vi "ALL1.vi"   [LabVIEW 2016, in "Test2.lvrbt"]
uses:
  Test2.lvrbt
  <vilib>/NXT/Hardware/Plugins/Tetrix DC Motor/TetrixDCMotorAddress.ctl
  <vilib>/NXT/Hardware/Plugins/Tetrix 180 deg Servo/Tetrix180ServoAddress.ctl
  <vilib>/NXT/Block Support/NXT_InputPort.ctl
  <vilib>/NXT/Subs/ColorSensorColors.ctl
  <vilib>/NXT/NXTIO Xnodes/NXTIONodeSubVIs/TETRIX IO Move Servos.vi
  <vilib>/NXT/Dual Mode Library/Waits/Wait_Num.vi
  <vilib>/NXT/NXTIO Xnodes/NXTIONodeSubVIs/TETRIX IO Move DC Motors.vi
  <vilib>/NXT/NXTIO Xnodes/NXTIONodeSubVIs/TETRIX IO Stop DC Motors.vi
  <vilib>/NXT/Dual Mode Library/Waits/Wait_EV3_Ultrasonic_Centimeter_Closer.vi
  <vilib>/NXT/Dual Mode Library/Waits/Wait_EV3_Ultrasonic_Centimeters_Further.vi
  <vilib>/NXT/Dual Mode Library/Waits/Wait_Touch.vi
  <vilib>/NXT/Dual Mode Library/Waits/Wait_EV3_Color_Color.vi
  <vilib>/NXT/NXTIO Xnodes/AddressXNode/NXTIOAddress.xnode
  <vilib>/NXT/Subs/LVHSConnector.ctl
  <vilib>/NXT/NXTIO Xnodes/NXTIOXNode/NXTIO.xnode
  <vilib>/NXT/LegoClasses/BrickReference/BrickReference.lvclass
types:
  T1 = typedef "Tetrix180ServoAddress.ctl" = i32
  T2 = cluster{"Tetrix180Servo":T1, "Tetrix180Servo 2":T1, "Tetrix180Servo 3":T1, "Tetrix180Servo 4":T1, "Tetrix180Servo 5":T1, "Tetrix180Servo 6":T1}
  T3 = typedef "TetrixDCMotorAddress.ctl" = i32
  T4 = cluster{"TetrixDCMotor":T3, "TetrixDCMotor 2":T3}
  T5 = cluster{"Tetrix180Servo":T1, "Tetrix180Servo":T1, "Tetrix180Servo":T1, "Tetrix180Servo":T1, "Tetrix180Servo":T1, "Tetrix180Servo":T1}
  T6 = typedef "LVHSConnector.ctl" = refnum<class "BrickReference.lvclass">
  T7 = typedef "NXT_InputPort.ctl" = u32
  T8 = typedef "ColorSensorColors.ctl" = enum16{"No Color", "Black", "Blue", "Green", "Yellow", "Red", "White", "Brown"}
diagram:
  # "FILE: BACK TOBASE2\n\nTHE ROBOT WILL GO TO BASE"
  # "FILE: SAVETOUCH \n\nTHE ROBOT WILL DETECT THE RACK \nAND STRAIGHT THE POSITION"
  # "FILE: SAVETOUCH \n\nTHE ROBOT WILL DETECT THE RACK \nAND STRAIGHT THE POSITION"
  # "FILE: DETECT REFERENCE LINE, AFTER AIMING\n\nTHE ROBOT WILL GET A NEW POSITION AFTER LAUNCH THE BALL"
  # "FILE: LAUNCHFIRSTBALL\n\nTHE SECOND BALL WILL BE  LAUNCH"
  # "FILE: TRAPBALL\n\nTHE ROBOT WILL MOVE FOWARD TO TRAP THE BALL"
  # "FILE: GETSEECONDBALL\n\nTHE ROBOT WILL START TO DETECT AND PICKUP THE SECOND BALL"
  # "FILE: DETECT REFERENCE LINE, AFTER AIMING\n\nTHE ROBOT WILL GET A NEW POSITION AFTER LAUNCH THE BALL"
  # "FILE: LAUNCHFIRSTBALL\n\nTHE FIRST BALL WILL BE  LAUNCH"
  # "FILE: SERVOSETTING\n\nTHE FIRST BALL WILL BE PICKUP"
  # "FILE: DETECTFIRSTBALL\n\nTHE ROBOT WILL MOVE INFRONT TO DETECT THE FIRST BALL"
  # "FILE: SAVETOUCH \n\nTHE ROBOT WILL DETECT THE RACK \nAND STRAIGHT THE POSITION"
  # "FILE:  motor setting\n\nTHE ROBOT WILL MOVE OUT FROM THE BASE."
  n1 = flat-sequence {
    tunnel: [w13] -> w12
    frame #0 {
      n2 = xnode "Motors"() -> ("Motor"=w22:T5)
      n3 = xnode "Move Servos"("Position 6"=u8 8, "Position 5"=u8 237, "Position 4"=u8 40, "Position 3"=u8 7, "Position 2"=u8 0, "Position 1"=u8 220, "Motors"=w22) -> ("NXT/EV3"=w15:T6)  [unwired: 1 in]
      n4 = xnode "Motors"() -> ("Motor"=w27:cluster{"TetrixDCMotor":T3, "TetrixDCMotor":T3})
      n5 = call-poly <vilib>:"PolyWait.vi"("Time (1 sec)"=sgl 1.0, "NXT/EV3"=w15) -> ("NXT/EV3"=w14:T6)  [unwired: 2 in]
      n6 = xnode "Move Motors"("Power/Speed 2"=i8 50, "Power/Speed 1"=i8 51, "Motors"=w27, "NXT/EV3"=w14) -> ("NXT/EV3"=w30:T6)
      n7 = call-poly <vilib>:"PolyWait.vi"("Time (1 sec)"=sgl 2.0, "NXT/EV3"=w30) -> ("NXT/EV3"=w28:T6)  [unwired: 2 in]
      n8 = xnode "Motors"() -> ("Motor"=w33:cluster{"TetrixDCMotor":T3, "TetrixDCMotor":T3})
      n9 = xnode "Stop Motors"("Motors"=w27, "NXT/EV3"=w28) -> ("NXT/EV3"=w26:T6)
      n10 = call-poly <vilib>:"PolyWait.vi"("Time (1 sec)"=sgl 1.0, "NXT/EV3"=w26) -> ("NXT/EV3"=w24:T6)  [unwired: 2 in]
      n11 = xnode "Move Motors"("Power/Speed 2"=i8 50, "Power/Speed 1"=i8 50, "Motors"=w33, "NXT/EV3"=w24) -> ("NXT/EV3"=w36:T6)
      n12 = call-poly <vilib>:"PolyWait.vi"("Time (1 sec)"=sgl 1.5, "NXT/EV3"=w36) -> ("NXT/EV3"=w34:T6)  [unwired: 2 in]
      n13 = xnode "Stop Motors"("Motors"=w33, "NXT/EV3"=w34) -> ("NXT/EV3"=w13:T6)
    }
  }
  n14 = flat-sequence {
    tunnel: w12 -> [w82]
    tunnel: [w81] -> w11
    frame #0 {
      w97 = T7 1 items=["Port 1", "Port 2", "Port 3", "Port 4"] ("Port (Port 1)")
      w113 = T7 1 items=["Port 1", "Port 2", "Port 3", "Port 4"] ("Port (Port 1)")
      n15 = xnode "Motors"() -> ("Motor"=w126:cluster{"TetrixDCMotor":T3, "TetrixDCMotor":T3})
      n16 = call-poly <vilib>:"PolyWait.vi"("Time (1 sec)"=sgl 1.0, "NXT/EV3"=w82) -> ("NXT/EV3"=w83:T6)  [unwired: 2 in]
      n17 = xnode "Move Motors"("Power/Speed 2"=i8 50, "Power/Speed 1"=i8 50, "Motors"=w126, "NXT/EV3"=w83) -> ("NXT/EV3"=w129:T6)
      n18 = call-poly <vilib>:"PolyWait.vi"("Centimeters (40)"=sgl 8.0, "NXT/EV3"=w129, "Port (Port 1)"=w113) -> ("NXT/EV3"=w127:T6)  [unwired: 1 in]
      n19 = xnode "Motors"() -> ("Motor"=w94:cluster{"TetrixDCMotor":T3, "TetrixDCMotor":T3})
      n20 = xnode "Stop Motors"("Motors"=w126, "NXT/EV3"=w127) -> ("NXT/EV3"=w103:T6)
      n21 = call-poly <vilib>:"PolyWait.vi"("Time (1 sec)"=sgl 1.0, "NXT/EV3"=w103) -> ("NXT/EV3"=w86:T6)  [unwired: 2 in]
      n22 = xnode "Move Motors"("Power/Speed 2"=i8 -5, "Power/Speed 1"=i8 -5, "Motors"=w94, "NXT/EV3"=w86) -> ("NXT/EV3"=w100:T6)
      n23 = call-poly <vilib>:"PolyWait.vi"("Centimeters (50)"=sgl 6.0, "NXT/EV3"=w100, "Port (Port 1)"=w97) -> ("NXT/EV3"=w98:T6)  [unwired: 1 in]
      n24 = xnode "Motors"() -> ("Motor"=w88:cluster{"TetrixDCMotor":T3, "TetrixDCMotor":T3})
      n25 = xnode "Stop Motors"("Motors"=w94, "NXT/EV3"=w98) -> ("NXT/EV3"=w92:T6)
      n26 = call-poly <vilib>:"PolyWait.vi"("Time (1 sec)"=sgl 1.0, "NXT/EV3"=w92) -> ("NXT/EV3"=w91:T6)  [unwired: 2 in]
      n27 = xnode "Move Motors"("Power/Speed 2"=i8 5, "Power/Speed 1"=i8 5, "Motors"=w88, "NXT/EV3"=w91) -> ("NXT/EV3"=w90:T6)
      n28 = call-poly <vilib>:"PolyWait.vi"("Time (1 sec)"=sgl 1.0, "NXT/EV3"=w90) -> ("NXT/EV3"=w89:T6)  [unwired: 2 in]
      n29 = xnode "Motors"() -> ("Motor"=w122:T3)
      n30 = xnode "Motors"() -> ("Motor"=w118:T3)
      n31 = xnode "Stop Motors"("Motors"=w88, "NXT/EV3"=w89) -> ("NXT/EV3"=w85:T6)
      n32 = call-poly <vilib>:"PolyWait.vi"("Time (1 sec)"=sgl 1.5, "NXT/EV3"=w85) -> ("NXT/EV3"=w116:T6)  [unwired: 2 in]
      n33 = xnode "Motors"() -> ("Sensor"=w115:T7)
      n34 = xnode "Motors"() -> ("Sensor"=w114:T7)
      n35 = xnode "Move Motors"("Power/Speed 1"=i8 10, "Motors"=w122, "NXT/EV3"=w116) -> ("NXT/EV3"=w124:T6)
      n36 = xnode "Move Motors"("Power/Speed 1"=i8 10, "Motors"=w118, "NXT/EV3"=w116) -> ("NXT/EV3"=w119:T6)
      n37 = call-poly <vilib>:"PolyWait.vi"("NXT/EV3"=w124, "Port (Port 1)"=w114) -> ("NXT/EV3"=w123:T6)  [unwired: 2 in]
      n38 = call-poly <vilib>:"PolyWait.vi"("NXT/EV3"=w119, "Port (Port 1)"=w115) -> ("NXT/EV3"=w117:T6)  [unwired: 2 in]
      n39 = xnode "Motors"() -> ("Motor"=w80:cluster{"TetrixDCMotor":T3, "TetrixDCMotor":T3})
      n40 = xnode "Stop Motors"("Motors"=w122, "NXT/EV3"=w123) -> ()  [unwired: 1 out]
      n41 = xnode "Stop Motors"("Motors"=w118, "NXT/EV3"=w117) -> ("NXT/EV3"=w112:T6)
      n42 = call-poly <vilib>:"PolyWait.vi"("Time (1 sec)"=sgl 2.0, "NXT/EV3"=w112) -> ("NXT/EV3"=w109:T6)  [unwired: 2 in]
      n43 = xnode "Move Motors"("Power/Speed 2"=i8 -5, "Power/Speed 1"=i8 -5, "Motors"=w80, "NXT/EV3"=w109) -> ("NXT/EV3"=w106:T6)
      n44 = call-poly <vilib>:"PolyWait.vi"("Time (1 sec)"=sgl 0.2, "NXT/EV3"=w106) -> ("NXT/EV3"=w105:T6)  [unwired: 2 in]
      n45 = xnode "Stop Motors"("Motors"=w80, "NXT/EV3"=w105) -> ("NXT/EV3"=w81:T6)
    }
  }
  n46 = flat-sequence {
    tunnel: w11 -> [w217]
    tunnel: [w216] -> w10
    frame #0 {
      w232 = T7 1 items=["Port 1", "Port 2", "Port 3", "Port 4"] ("Port (Port 1)")
      n47 = xnode "Motors"() -> ("Motor"=w228:cluster{"TetrixDCMotor":T3, "TetrixDCMotor":T3})
      n48 = call-poly <vilib>:"PolyWait.vi"("Time (1 sec)"=sgl 1.0, "NXT/EV3"=w217) -> ("NXT/EV3"=w229:T6)  [unwired: 2 in]
      n49 = xnode "Move Motors"("Power/Speed 2"=i8 20, "Power/Speed 1"=i8 20, "Motors"=w228, "NXT/EV3"=w229) -> ("NXT/EV3"=w235:T6)
      n50 = call-poly <vilib>:"PolyWait.vi"("Centimeters (50)"=sgl 6.0, "NXT/EV3"=w235, "Port (Port 1)"=w232) -> ("NXT/EV3"=w233:T6)  [unwired: 1 in]
      n51 = xnode "Motors"() -> ("Motor"=w224:cluster{"TetrixDCMotor":T3, "TetrixDCMotor":T3})
      n52 = xnode "Stop Motors"("Motors"=w228, "NXT/EV3"=w233) -> ("NXT/EV3"=w218:T6)
      n53 = call-poly <vilib>:"PolyWait.vi"("Time (1 sec)"=sgl 1.0, "NXT/EV3"=w218) -> ("NXT/EV3"=w219:T6)  [unwired: 2 in]
      n54 = xnode "Motors"() -> ("Sensor"=w221:T7)
      n55 = xnode "Move Motors"("Power/Speed 2"=i8 -5, "Power/Speed 1"=i8 -5, "Motors"=w224, "NXT/EV3"=w219) -> ("NXT/EV3"=w226:T6)
      n56 = call-poly <vilib>:"PolyWait.vi"("Centimeters (40)"=sgl 11.0 ("Centimeters (50)"), "NXT/EV3"=w226, "Port (Port 1)"=w221) -> ("NXT/EV3"=w225:T6)  [unwired: 1 in]
      n57 = xnode "Stop Motors"("Motors"=w224, "NXT/EV3"=w225) -> ("NXT/EV3"=w216:T6)
    }
  }
  n58 = flat-sequence {
    tunnel: w10 -> [w267]
    tunnel: [w266] -> w9
    frame #0 {
      n59 = xnode "Motors"() -> ("Motor"=w272:T1)
      n60 = call-poly <vilib>:"PolyWait.vi"("Time (1 sec)"=sgl 1.0, "NXT/EV3"=w267) -> ("NXT/EV3"=w269:T6)  [unwired: 2 in]
      n61 = xnode "Move Servos"("Position 1"=u8 124, "Motors"=w272, "NXT/EV3"=w269) -> ("NXT/EV3"=w270:T6)
      n62 = xnode "Motors"() -> ("Motor"=w301:T1)
      n63 = call-poly <vilib>:"PolyWait.vi"("Time (1 sec)"=sgl 1.0, "NXT/EV3"=w270) -> ("NXT/EV3"=w283:T6)  [unwired: 2 in]
      n64 = xnode "Move Servos"("Position 1"=u8 70, "Motors"=w301, "NXT/EV3"=w283) -> ("NXT/EV3"=w298:T6)
      n65 = xnode "Motors"() -> ("Motor"=w297:T1)
      n66 = call-poly <vilib>:"PolyWait.vi"("Time (1 sec)"=sgl 7.0, "NXT/EV3"=w298) -> ("NXT/EV3"=w295:T6)  [unwired: 2 in]
      n67 = xnode "Move Servos"("Position 1"=u8 227, "Motors"=w297, "NXT/EV3"=w295) -> ("NXT/EV3"=w293:T6)
      n68 = xnode "Motors"() -> ("Motor"=w292:T1)
      n69 = call-poly <vilib>:"PolyWait.vi"("Time (1 sec)"=sgl 0.5, "NXT/EV3"=w293) -> ("NXT/EV3"=w290:T6)  [unwired: 2 in]
      n70 = xnode "Move Servos"("Position 1"=u8 8, "Motors"=w292, "NXT/EV3"=w290) -> ("NXT/EV3"=w288:T6)
      n71 = xnode "Motors"() -> ("Motor"=w286:T1)
      n72 = call-poly <vilib>:"PolyWait.vi"("Time (1 sec)"=sgl 1.0, "NXT/EV3"=w288) -> ("NXT/EV3"=w285:T6)  [unwired: 2 in]
      n73 = xnode "Move Servos"("Position 1"=u8 82, "Motors"=w286, "NXT/EV3"=w285) -> ("NXT/EV3"=w268:T6)
      n74 = xnode "Motors"() -> ("Motor"=w280:T1)
      n75 = call-poly <vilib>:"PolyWait.vi"("Time (1 sec)"=sgl 1.0, "NXT/EV3"=w268) -> ("NXT/EV3"=w279:T6)  [unwired: 2 in]
      n76 = xnode "Move Servos"("Position 1"=u8 67, "Motors"=w280, "NXT/EV3"=w279) -> ("NXT/EV3"=w277:T6)
      n77 = xnode "Motors"() -> ("Motor"=w275:T1)
      n78 = call-poly <vilib>:"PolyWait.vi"("Time (1 sec)"=sgl 1.0, "NXT/EV3"=w277) -> ("NXT/EV3"=w274:T6)  [unwired: 2 in]
      n79 = xnode "Move Servos"("Position 1"=u8 240, "Motors"=w275, "NXT/EV3"=w274) -> ("NXT/EV3"=w266:T6)
    }
  }
  n80 = flat-sequence {
    tunnel: w9 -> [w359]
    tunnel: [w358] -> w8
    frame #0 {
      n81 = xnode "Motors"() -> ("Motor"=w396:T1)
      n82 = call-poly <vilib>:"PolyWait.vi"("Time (1 sec)"=sgl 1.0, "NXT/EV3"=w359) -> ("NXT/EV3"=w360:T6)  [unwired: 2 in]
      n83 = xnode "Move Servos"("Position 1"=u8 255, "Motors"=w396, "NXT/EV3"=w360) -> ("NXT/EV3"=w393:T6)
      n84 = xnode "Motors"() -> ("Motor"=w397:cluster{"TetrixDCMotor":T3, "TetrixDCMotor":T3})
      n85 = call-poly <vilib>:"PolyWait.vi"("Time (1 sec)"=sgl 1.0, "NXT/EV3"=w393) -> ("NXT/EV3"=w392:T6)  [unwired: 2 in]
      n86 = xnode "Move Motors"("Power/Speed 2"=i8 -50, "Power/Speed 1"=i8 -50, "Motors"=w397, "NXT/EV3"=w392) -> ("NXT/EV3"=w400:T6)
      n87 = call-poly <vilib>:"PolyWait.vi"("Time (1 sec)"=sgl 0.5, "NXT/EV3"=w400) -> ("NXT/EV3"=w398:T6)  [unwired: 2 in]
      n88 = xnode "Motors"() -> ("Motor"=w388:T1)
      n89 = xnode "Stop Motors"("Motors"=w397, "NXT/EV3"=w398) -> ("NXT/EV3"=w391:T6)
      n90 = call-poly <vilib>:"PolyWait.vi"("Time (1 sec)"=sgl 1.0, "NXT/EV3"=w391) -> ("NXT/EV3"=w389:T6)  [unwired: 2 in]
      n91 = xnode "Move Servos"("Position 1"=u8 0, "Motors"=w388, "NXT/EV3"=w389) -> ("NXT/EV3"=w382:T6)
      n92 = xnode "Motors"() -> ("Motor"=w384:T1)
      n93 = call-poly <vilib>:"PolyWait.vi"("Time (1 sec)"=sgl 1.0, "NXT/EV3"=w382) -> ("NXT/EV3"=w385:T6)  [unwired: 2 in]
      n94 = xnode "Move Servos"("Position 1"=u8 230, "Motors"=w384, "NXT/EV3"=w385) -> ("NXT/EV3"=w377:T6)
      n95 = xnode "Motors"() -> ("Motor"=w379:T1)
      n96 = call-poly <vilib>:"PolyWait.vi"("Time (1 sec)"=sgl 1.0, "NXT/EV3"=w377) -> ("NXT/EV3"=w380:T6)  [unwired: 2 in]
      n97 = xnode "Move Servos"("Position 1"=u8 7, "Motors"=w379, "NXT/EV3"=w380) -> ("NXT/EV3"=w372:T6)
      n98 = xnode "Motors"() -> ("Motor"=w374:T1)
      n99 = call-poly <vilib>:"PolyWait.vi"("Time (1 sec)"=sgl 0.5, "NXT/EV3"=w372) -> ("NXT/EV3"=w375:T6)  [unwired: 2 in]
      n100 = xnode "Move Servos"("Position 1"=u8 220, "Motors"=w374, "NXT/EV3"=w375) -> ("NXT/EV3"=w367:T6)
      n101 = xnode "Motors"() -> ("Motor"=w369:T1)
      n102 = call-poly <vilib>:"PolyWait.vi"("Time (1 sec)"=sgl 1.0, "NXT/EV3"=w367) -> ("NXT/EV3"=w370:T6)  [unwired: 2 in]
      n103 = xnode "Move Servos"("Position 1"=u8 114, "Motors"=w369, "NXT/EV3"=w370) -> ("NXT/EV3"=w362:T6)
      n104 = xnode "Motors"() -> ("Motor"=w364:T1)
      n105 = call-poly <vilib>:"PolyWait.vi"("Time (1 sec)"=sgl 1.5, "NXT/EV3"=w362) -> ("NXT/EV3"=w365:T6)  [unwired: 2 in]
      n106 = xnode "Move Servos"("Position 1"=u8 40, "Motors"=w364, "NXT/EV3"=w365) -> ("NXT/EV3"=w358:T6)
    }
  }
  n107 = flat-sequence {
    tunnel: w8 -> [w484]
    tunnel: [w473] -> w7
    frame #0 {
      w487 = T7 2 items=["Port 1", "Port 2", "Port 3", "Port 4"] ("Port (Port 1)")
      w496 = T7 2 items=["Port 1", "Port 2", "Port 3", "Port 4"] ("Port (Port 1)")
      n108 = xnode "Motors"() -> ("Motor"=w506:cluster{"TetrixDCMotor":T3, "TetrixDCMotor":T3})
      n109 = call-poly <vilib>:"PolyWait.vi"("Time (1 sec)"=sgl 16.0, "NXT/EV3"=w484) -> ("NXT/EV3"=w483:T6)  [unwired: 2 in]
      n110 = xnode "Move Motors"("Power/Speed 2"=i8 -50, "Power/Speed 1"=i8 -50, "Motors"=w506, "NXT/EV3"=w483) -> ("NXT/EV3"=w509:T6)
      n111 = call-poly <vilib>:"PolyWait.vi"("Time (1 sec)"=sgl 0.5, "NXT/EV3"=w509) -> ("NXT/EV3"=w508:T6)  [unwired: 2 in]
      n112 = xnode "Motors"() -> ("Motor"=w501:cluster{"TetrixDCMotor":T3, "TetrixDCMotor":T3})
      n113 = xnode "Stop Motors"("Motors"=w506, "NXT/EV3"=w508) -> ("NXT/EV3"=w499:T6)
      n114 = call-poly <vilib>:"PolyWait.vi"("Time (1 sec)"=sgl 1.0, "NXT/EV3"=w499) -> ("NXT/EV3"=w498:T6)  [unwired: 2 in]
      n115 = xnode "Move Motors"("Power/Speed 2"=i8 20, "Power/Speed 1"=i8 20, "Motors"=w501, "NXT/EV3"=w498) -> ("NXT/EV3"=w503:T6)
      n116 = call-poly <vilib>:"PolyWait.vi"("Color (Red)"=ColorSensorColors."Black", "NXT/EV3"=w503, "Port (Port 1)"=w496) -> ("NXT/EV3"=w502:T6)  [unwired: 1 in]
      n117 = xnode "Motors"() -> ("Motor"=w491:cluster{"TetrixDCMotor":T3, "TetrixDCMotor":T3})
      n118 = xnode "Stop Motors"("Motors"=w501, "NXT/EV3"=w502) -> ("NXT/EV3"=w486:T6)
      n119 = call-poly <vilib>:"PolyWait.vi"("Time (1 sec)"=sgl 0.5, "NXT/EV3"=w486) -> ("NXT/EV3"=w489:T6)  [unwired: 2 in]
      n120 = xnode "Move Motors"("Power/Speed 2"=i8 -20, "Power/Speed 1"=i8 -20, "Motors"=w491, "NXT/EV3"=w489) -> ("NXT/EV3"=w493:T6)
      n121 = call-poly <vilib>:"PolyWait.vi"("Color (Red)"=ColorSensorColors."Black", "NXT/EV3"=w493, "Port (Port 1)"=w487) -> ("NXT/EV3"=w492:T6)  [unwired: 1 in]
      n122 = xnode "Motors"() -> ("Motor"=w477:cluster{"TetrixDCMotor":T3, "TetrixDCMotor":T3})
      n123 = xnode "Stop Motors"("Motors"=w491, "NXT/EV3"=w492) -> ("NXT/EV3"=w475:T6)
      n124 = call-poly <vilib>:"PolyWait.vi"("Time (1 sec)"=sgl 0.5, "NXT/EV3"=w475) -> ("NXT/EV3"=w474:T6)  [unwired: 2 in]
      n125 = xnode "Move Motors"("Power/Speed 2"=i8 -5, "Power/Speed 1"=i8 -5, "Motors"=w477, "NXT/EV3"=w474) -> ("NXT/EV3"=w480:T6)
      n126 = call-poly <vilib>:"PolyWait.vi"("Time (1 sec)"=sgl 1.0, "NXT/EV3"=w480) -> ("NXT/EV3"=w479:T6)  [unwired: 2 in]
      n127 = xnode "Stop Motors"("Motors"=w477, "NXT/EV3"=w479) -> ("NXT/EV3"=w473:T6)
    }
  }
  n128 = flat-sequence {
    tunnel: w7 -> [w571]
    tunnel: [w569] -> w6
    frame #0 {
      w586 = T7 1 items=["Port 1", "Port 2", "Port 3", "Port 4"] ("Port (Port 1)")
      w613 = T7 1 items=["Port 1", "Port 2", "Port 3", "Port 4"] ("Port (Port 1)")
      n129 = xnode "Motors"() -> ("Motor"=w602:T5)
      n130 = call-poly <vilib>:"PolyWait.vi"("Time (1 sec)"=sgl 1.0, "NXT/EV3"=w571) -> ("NXT/EV3"=w572:T6)  [unwired: 2 in]
      n131 = xnode "Move Servos"("Position 6"=u8 8, "Position 5"=u8 237, "Position 4"=u8 40, "Position 3"=u8 7, "Position 2"=u8 0, "Position 1"=u8 220, "Motors"=w602, "NXT/EV3"=w572) -> ("NXT/EV3"=w595:T6)
      n132 = xnode "Motors"() -> ("Motor"=w626:cluster{"TetrixDCMotor":T3, "TetrixDCMotor":T3})
      n133 = call-poly <vilib>:"PolyWait.vi"("Time (1 sec)"=sgl 1.0, "NXT/EV3"=w595) -> ("NXT/EV3"=w594:T6)  [unwired: 2 in]
      n134 = xnode "Move Motors"("Power/Speed 2"=i8 50, "Power/Speed 1"=i8 50, "Motors"=w626, "NXT/EV3"=w594) -> ("NXT/EV3"=w629:T6)
      n135 = call-poly <vilib>:"PolyWait.vi"("Centimeters (40)"=sgl 8.0, "NXT/EV3"=w629, "Port (Port 1)"=w613) -> ("NXT/EV3"=w627:T6)  [unwired: 1 in]
      n136 = xnode "Motors"() -> ("Motor"=w583:cluster{"TetrixDCMotor":T3, "TetrixDCMotor":T3})
      n137 = xnode "Stop Motors"("Motors"=w626, "NXT/EV3"=w627) -> ("NXT/EV3"=w592:T6)
      n138 = call-poly <vilib>:"PolyWait.vi"("Time (1 sec)"=sgl 1.0, "NXT/EV3"=w592) -> ("NXT/EV3"=w575:T6)  [unwired: 2 in]
      n139 = xnode "Move Motors"("Power/Speed 2"=i8 -5, "Power/Speed 1"=i8 -5, "Motors"=w583, "NXT/EV3"=w575) -> ("NXT/EV3"=w589:T6)
      n140 = call-poly <vilib>:"PolyWait.vi"("Centimeters (50)"=sgl 6.0, "NXT/EV3"=w589, "Port (Port 1)"=w586) -> ("NXT/EV3"=w587:T6)  [unwired: 1 in]
      n141 = xnode "Motors"() -> ("Motor"=w577:cluster{"TetrixDCMotor":T3, "TetrixDCMotor":T3})
      n142 = xnode "Stop Motors"("Motors"=w583, "NXT/EV3"=w587) -> ("NXT/EV3"=w581:T6)
      n143 = call-poly <vilib>:"PolyWait.vi"("Time (1 sec)"=sgl 1.0, "NXT/EV3"=w581) -> ("NXT/EV3"=w580:T6)  [unwired: 2 in]
      n144 = xnode "Move Motors"("Power/Speed 2"=i8 5, "Power/Speed 1"=i8 5, "Motors"=w577, "NXT/EV3"=w580) -> ("NXT/EV3"=w579:T6)
      n145 = call-poly <vilib>:"PolyWait.vi"("Time (1 sec)"=sgl 1.0, "NXT/EV3"=w579) -> ("NXT/EV3"=w578:T6)  [unwired: 2 in]
      n146 = xnode "Motors"() -> ("Motor"=w622:T3)
      n147 = xnode "Motors"() -> ("Motor"=w618:T3)
      n148 = xnode "Stop Motors"("Motors"=w577, "NXT/EV3"=w578) -> ("NXT/EV3"=w574:T6)
      n149 = call-poly <vilib>:"PolyWait.vi"("Time (1 sec)"=sgl 1.5, "NXT/EV3"=w574) -> ("NXT/EV3"=w616:T6)  [unwired: 2 in]
      n150 = xnode "Motors"() -> ("Sensor"=w615:T7)
      n151 = xnode "Motors"() -> ("Sensor"=w614:T7)
      n152 = xnode "Move Motors"("Power/Speed 1"=i8 10, "Motors"=w622, "NXT/EV3"=w616) -> ("NXT/EV3"=w624:T6)
      n153 = xnode "Move Motors"("Power/Speed 1"=i8 10, "Motors"=w618, "NXT/EV3"=w616) -> ("NXT/EV3"=w619:T6)
      n154 = call-poly <vilib>:"PolyWait.vi"("NXT/EV3"=w624, "Port (Port 1)"=w614) -> ("NXT/EV3"=w623:T6)  [unwired: 2 in]
      n155 = call-poly <vilib>:"PolyWait.vi"("NXT/EV3"=w619, "Port (Port 1)"=w615) -> ("NXT/EV3"=w617:T6)  [unwired: 2 in]
      n156 = xnode "Motors"() -> ("Motor"=w610:cluster{"TetrixDCMotor":T3, "TetrixDCMotor":T3})
      n157 = xnode "Stop Motors"("Motors"=w622, "NXT/EV3"=w623) -> ()  [unwired: 1 out]
      n158 = xnode "Stop Motors"("Motors"=w618, "NXT/EV3"=w617) -> ("NXT/EV3"=w612:T6)
      n159 = call-poly <vilib>:"PolyWait.vi"("Time (1 sec)"=sgl 2.0, "NXT/EV3"=w612) -> ("NXT/EV3"=w608:T6)  [unwired: 2 in]
      n160 = xnode "Move Motors"("Power/Speed 2"=i8 -5, "Power/Speed 1"=i8 -5, "Motors"=w610, "NXT/EV3"=w608) -> ("NXT/EV3"=w605:T6)
      n161 = call-poly <vilib>:"PolyWait.vi"("Time (1 sec)"=sgl 0.2, "NXT/EV3"=w605) -> ("NXT/EV3"=w604:T6)  [unwired: 2 in]
      n162 = xnode "Stop Motors"("Motors"=w610, "NXT/EV3"=w604) -> ("NXT/EV3"=w568:T6)
      n163 = call-poly <vilib>:"PolyWait.vi"("Time (1 sec)"=sgl 1.0, "NXT/EV3"=w568) -> ("NXT/EV3"=w569:T6)  [unwired: 2 in]
    }
  }
  n164 = flat-sequence {
    tunnel: w6 -> [w730]
    tunnel: [w729] -> w5
    frame #0 {
      w778 = T7 1 items=["Port 1", "Port 2", "Port 3", "Port 4"] ("Port (Port 1)")
      n165 = xnode "Motors"() -> ("Motor"=w773:T5)
      n166 = xnode "Move Servos"("Position 6"=u8 8, "Position 5"=u8 237, "Position 4"=u8 40, "Position 3"=u8 7, "Position 2"=u8 0, "Position 1"=u8 220, "Motors"=w773, "NXT/EV3"=w730) -> ("NXT/EV3"=w766:T6)
      n167 = xnode "Motors"() -> ("Motor"=w774:cluster{"TetrixDCMotor":T3, "TetrixDCMotor":T3})
      n168 = call-poly <vilib>:"PolyWait.vi"("Time (1 sec)"=sgl 0.5, "NXT/EV3"=w766) -> ("NXT/EV3"=w775:T6)  [unwired: 2 in]
      n169 = xnode "Move Motors"("Power/Speed 2"=i8 20, "Power/Speed 1"=i8 20, "Motors"=w774, "NXT/EV3"=w775) -> ("NXT/EV3"=w781:T6)
      n170 = call-poly <vilib>:"PolyWait.vi"("Centimeters (50)"=sgl 6.0, "NXT/EV3"=w781, "Port (Port 1)"=w778) -> ("NXT/EV3"=w779:T6)  [unwired: 1 in]
      n171 = xnode "Motors"() -> ("Motor"=w761:cluster{"TetrixDCMotor":T3, "TetrixDCMotor":T3})
      n172 = xnode "Stop Motors"("Motors"=w774, "NXT/EV3"=w779) -> ("NXT/EV3"=w765:T6)
      n173 = call-poly <vilib>:"PolyWait.vi"("Time (1 sec)"=sgl 1.0, "NXT/EV3"=w765) -> ("NXT/EV3"=w756:T6)  [unwired: 2 in]
      n174 = xnode "Motors"() -> ("Sensor"=w758:T7)
      n175 = xnode "Move Motors"("Power/Speed 2"=i8 -5, "Power/Speed 1"=i8 -5, "Motors"=w761, "NXT/EV3"=w756) -> ("NXT/EV3"=w763:T6)
      n176 = call-poly <vilib>:"PolyWait.vi"("Centimeters (40)"=sgl 6.0 ("Centimeters (50)"), "NXT/EV3"=w763, "Port (Port 1)"=w758) -> ("NXT/EV3"=w762:T6)  [unwired: 1 in]
      n177 = xnode "Motors"() -> ("Motor"=w735:T1)
      n178 = xnode "Stop Motors"("Motors"=w761, "NXT/EV3"=w762) -> ("NXT/EV3"=w731:T6)
      n179 = call-poly <vilib>:"PolyWait.vi"("Time (1 sec)"=sgl 1.0, "NXT/EV3"=w731) -> ("NXT/EV3"=w732:T6)  [unwired: 2 in]
      n180 = xnode "Move Servos"("Position 1"=u8 124, "Motors"=w735, "NXT/EV3"=w732) -> ("NXT/EV3"=w733:T6)
      n181 = xnode "Motors"() -> ("Motor"=w755:T1)
      n182 = call-poly <vilib>:"PolyWait.vi"("Time (1 sec)"=sgl 1.0, "NXT/EV3"=w733) -> ("NXT/EV3"=w737:T6)  [unwired: 2 in]
      n183 = xnode "Move Servos"("Position 1"=u8 70, "Motors"=w755, "NXT/EV3"=w737) -> ("NXT/EV3"=w752:T6)
      n184 = xnode "Motors"() -> ("Motor"=w751:T1)
      n185 = call-poly <vilib>:"PolyWait.vi"("Time (1 sec)"=sgl 7.0, "NXT/EV3"=w752) -> ("NXT/EV3"=w749:T6)  [unwired: 2 in]
      n186 = xnode "Move Servos"("Position 1"=u8 227, "Motors"=w751, "NXT/EV3"=w749) -> ("NXT/EV3"=w747:T6)
      n187 = xnode "Motors"() -> ("Motor"=w746:T1)
      n188 = call-poly <vilib>:"PolyWait.vi"("Time (1 sec)"=sgl 0.5, "NXT/EV3"=w747) -> ("NXT/EV3"=w744:T6)  [unwired: 2 in]
      n189 = xnode "Move Servos"("Position 1"=u8 8, "Motors"=w746, "NXT/EV3"=w744) -> ("NXT/EV3"=w742:T6)
      n190 = xnode "Motors"() -> ("Motor"=w740:T1)
      n191 = call-poly <vilib>:"PolyWait.vi"("Time (1 sec)"=sgl 1.0, "NXT/EV3"=w742) -> ("NXT/EV3"=w739:T6)  [unwired: 2 in]
      n192 = xnode "Move Servos"("Position 1"=u8 82, "Motors"=w740, "NXT/EV3"=w739) -> ("NXT/EV3"=w729:T6)
    }
  }
  n193 = flat-sequence {
    tunnel: w5 -> [w866]
    tunnel: [w865] -> w4
    frame #0 {
      w882 = T7 1 items=["Port 1", "Port 2", "Port 3", "Port 4"] ("Port (Port 1)")
      n194 = xnode "Motors"() -> ("Motor"=w879:cluster{"TetrixDCMotor":T3, "TetrixDCMotor":T3})
      n195 = call-poly <vilib>:"PolyWait.vi"("Time (1 sec)"=sgl 1.0, "NXT/EV3"=w866) -> ("NXT/EV3"=w877:T6)  [unwired: 2 in]
      n196 = xnode "Move Motors"("Power/Speed 1"=i8 20, "Motors"=w879, "NXT/EV3"=w877, "Power/Speed 2"=i8 20) -> ("NXT/EV3"=w885:T6)
      n197 = call-poly <vilib>:"PolyWait.vi"("Centimeters (50)"=sgl 6.0, "NXT/EV3"=w885, "Port (Port 1)"=w882) -> ("NXT/EV3"=w883:T6)  [unwired: 1 in]
      n198 = xnode "Motors"() -> ("Motor"=w874:T1)
      n199 = xnode "Stop Motors"("Motors"=w879, "NXT/EV3"=w883) -> ("NXT/EV3"=w867:T6)
      n200 = call-poly <vilib>:"PolyWait.vi"("Time (1 sec)"=sgl 1.0, "NXT/EV3"=w867) -> ("NXT/EV3"=w873:T6)  [unwired: 2 in]
      n201 = xnode "Move Servos"("Position 1"=u8 67, "Motors"=w874, "NXT/EV3"=w873) -> ("NXT/EV3"=w871:T6)
      n202 = xnode "Motors"() -> ("Motor"=w869:T1)
      n203 = call-poly <vilib>:"PolyWait.vi"("Time (1 sec)"=sgl 1.0, "NXT/EV3"=w871) -> ("NXT/EV3"=w868:T6)  [unwired: 2 in]
      n204 = xnode "Move Servos"("Position 1"=u8 240, "Motors"=w869, "NXT/EV3"=w868) -> ("NXT/EV3"=w865:T6)
    }
  }
  n205 = flat-sequence {
    tunnel: [w917] -> w3
    tunnel: w4 -> [w916]
    frame #0 {
      n206 = xnode "Motors"() -> ("Motor"=w954:T1)
      n207 = call-poly <vilib>:"PolyWait.vi"("Time (1 sec)"=sgl 1.0, "NXT/EV3"=w916) -> ("NXT/EV3"=w918:T6)  [unwired: 2 in]
      n208 = xnode "Move Servos"("Position 1"=u8 255, "Motors"=w954, "NXT/EV3"=w918) -> ("NXT/EV3"=w951:T6)
      n209 = xnode "Motors"() -> ("Motor"=w955:cluster{"TetrixDCMotor":T3, "TetrixDCMotor":T3})
      n210 = call-poly <vilib>:"PolyWait.vi"("Time (1 sec)"=sgl 1.0, "NXT/EV3"=w951) -> ("NXT/EV3"=w950:T6)  [unwired: 2 in]
      n211 = xnode "Move Motors"("Power/Speed 2"=i8 -50, "Power/Speed 1"=i8 -50, "Motors"=w955, "NXT/EV3"=w950) -> ("NXT/EV3"=w958:T6)
      n212 = call-poly <vilib>:"PolyWait.vi"("Time (1 sec)"=sgl 0.5, "NXT/EV3"=w958) -> ("NXT/EV3"=w956:T6)  [unwired: 2 in]
      n213 = xnode "Motors"() -> ("Motor"=w946:T1)
      n214 = xnode "Stop Motors"("Motors"=w955, "NXT/EV3"=w956) -> ("NXT/EV3"=w949:T6)
      n215 = call-poly <vilib>:"PolyWait.vi"("Time (1 sec)"=sgl 1.0, "NXT/EV3"=w949) -> ("NXT/EV3"=w947:T6)  [unwired: 2 in]
      n216 = xnode "Move Servos"("Position 1"=u8 0, "Motors"=w946, "NXT/EV3"=w947) -> ("NXT/EV3"=w940:T6)
      n217 = xnode "Motors"() -> ("Motor"=w942:T1)
      n218 = call-poly <vilib>:"PolyWait.vi"("Time (1 sec)"=sgl 1.0, "NXT/EV3"=w940) -> ("NXT/EV3"=w943:T6)  [unwired: 2 in]
      n219 = xnode "Move Servos"("Position 1"=u8 230, "Motors"=w942, "NXT/EV3"=w943) -> ("NXT/EV3"=w935:T6)
      n220 = xnode "Motors"() -> ("Motor"=w937:T1)
      n221 = call-poly <vilib>:"PolyWait.vi"("Time (1 sec)"=sgl 1.0, "NXT/EV3"=w935) -> ("NXT/EV3"=w938:T6)  [unwired: 2 in]
      n222 = xnode "Move Servos"("Position 1"=u8 7, "Motors"=w937, "NXT/EV3"=w938) -> ("NXT/EV3"=w930:T6)
      n223 = xnode "Motors"() -> ("Motor"=w932:T1)
      n224 = call-poly <vilib>:"PolyWait.vi"("Time (1 sec)"=sgl 0.5, "NXT/EV3"=w930) -> ("NXT/EV3"=w933:T6)  [unwired: 2 in]
      n225 = xnode "Move Servos"("Position 1"=u8 220, "Motors"=w932, "NXT/EV3"=w933) -> ("NXT/EV3"=w925:T6)
      n226 = xnode "Motors"() -> ("Motor"=w927:T1)
      n227 = call-poly <vilib>:"PolyWait.vi"("Time (1 sec)"=sgl 1.0, "NXT/EV3"=w925) -> ("NXT/EV3"=w928:T6)  [unwired: 2 in]
      n228 = xnode "Move Servos"("Position 1"=u8 114, "Motors"=w927, "NXT/EV3"=w928) -> ("NXT/EV3"=w920:T6)
      n229 = xnode "Motors"() -> ("Motor"=w922:T1)
      n230 = call-poly <vilib>:"PolyWait.vi"("Time (1 sec)"=sgl 1.5, "NXT/EV3"=w920) -> ("NXT/EV3"=w923:T6)  [unwired: 2 in]
      n231 = xnode "Move Servos"("Position 1"=u8 40, "Motors"=w922, "NXT/EV3"=w923) -> ("NXT/EV3"=w917:T6)
    }
  }
  n232 = flat-sequence {
    tunnel: w3 -> [w1042]
    tunnel: [w1031] -> w2
    frame #0 {
      w1045 = T7 2 items=["Port 1", "Port 2", "Port 3", "Port 4"] ("Port (Port 1)")
      w1054 = T7 2 items=["Port 1", "Port 2", "Port 3", "Port 4"] ("Port (Port 1)")
      n233 = xnode "Motors"() -> ("Motor"=w1064:cluster{"TetrixDCMotor":T3, "TetrixDCMotor":T3})
      n234 = call-poly <vilib>:"PolyWait.vi"("Time (1 sec)"=sgl 16.0, "NXT/EV3"=w1042) -> ("NXT/EV3"=w1041:T6)  [unwired: 2 in]
      n235 = xnode "Move Motors"("Power/Speed 2"=i8 -50, "Power/Speed 1"=i8 -50, "Motors"=w1064, "NXT/EV3"=w1041) -> ("NXT/EV3"=w1067:T6)
      n236 = call-poly <vilib>:"PolyWait.vi"("Time (1 sec)"=sgl 0.5, "NXT/EV3"=w1067) -> ("NXT/EV3"=w1066:T6)  [unwired: 2 in]
      n237 = xnode "Motors"() -> ("Motor"=w1059:cluster{"TetrixDCMotor":T3, "TetrixDCMotor":T3})
      n238 = xnode "Stop Motors"("Motors"=w1064, "NXT/EV3"=w1066) -> ("NXT/EV3"=w1057:T6)
      n239 = call-poly <vilib>:"PolyWait.vi"("Time (1 sec)"=sgl 1.0, "NXT/EV3"=w1057) -> ("NXT/EV3"=w1056:T6)  [unwired: 2 in]
      n240 = xnode "Move Motors"("Power/Speed 2"=i8 20, "Power/Speed 1"=i8 20, "Motors"=w1059, "NXT/EV3"=w1056) -> ("NXT/EV3"=w1061:T6)
      n241 = call-poly <vilib>:"PolyWait.vi"("Color (Red)"=ColorSensorColors."Black", "NXT/EV3"=w1061, "Port (Port 1)"=w1054) -> ("NXT/EV3"=w1060:T6)  [unwired: 1 in]
      n242 = xnode "Motors"() -> ("Motor"=w1049:cluster{"TetrixDCMotor":T3, "TetrixDCMotor":T3})
      n243 = xnode "Stop Motors"("Motors"=w1059, "NXT/EV3"=w1060) -> ("NXT/EV3"=w1044:T6)
      n244 = call-poly <vilib>:"PolyWait.vi"("Time (1 sec)"=sgl 0.5, "NXT/EV3"=w1044) -> ("NXT/EV3"=w1047:T6)  [unwired: 2 in]
      n245 = xnode "Move Motors"("Power/Speed 2"=i8 -20, "Power/Speed 1"=i8 -20, "Motors"=w1049, "NXT/EV3"=w1047) -> ("NXT/EV3"=w1051:T6)
      n246 = call-poly <vilib>:"PolyWait.vi"("Color (Red)"=ColorSensorColors."Black", "NXT/EV3"=w1051, "Port (Port 1)"=w1045) -> ("NXT/EV3"=w1050:T6)  [unwired: 1 in]
      n247 = xnode "Motors"() -> ("Motor"=w1035:cluster{"TetrixDCMotor":T3, "TetrixDCMotor":T3})
      n248 = xnode "Stop Motors"("Motors"=w1049, "NXT/EV3"=w1050) -> ("NXT/EV3"=w1033:T6)
      n249 = call-poly <vilib>:"PolyWait.vi"("Time (1 sec)"=sgl 0.5, "NXT/EV3"=w1033) -> ("NXT/EV3"=w1032:T6)  [unwired: 2 in]
      n250 = xnode "Move Motors"("Power/Speed 2"=i8 -5, "Power/Speed 1"=i8 -5, "Motors"=w1035, "NXT/EV3"=w1032) -> ("NXT/EV3"=w1038:T6)
      n251 = call-poly <vilib>:"PolyWait.vi"("Time (1 sec)"=sgl 1.0, "NXT/EV3"=w1038) -> ("NXT/EV3"=w1037:T6)  [unwired: 2 in]
      n252 = xnode "Stop Motors"("Motors"=w1035, "NXT/EV3"=w1037) -> ("NXT/EV3"=w1031:T6)
    }
  }
  n253 = flat-sequence {
    tunnel: [w1137] -> w1
    tunnel: w2 -> [w1126]
    frame #0 {
      w1152 = T7 1 items=["Port 1", "Port 2", "Port 3", "Port 4"] ("Port (Port 1)")
      w1169 = T7 1 items=["Port 1", "Port 2", "Port 3", "Port 4"] ("Port (Port 1)")
      n254 = xnode "Motors"() -> ("Motor"=w1136:T5)
      n255 = call-poly <vilib>:"PolyWait.vi"("Time (1 sec)"=sgl 1.0, "NXT/EV3"=w1126) -> ("NXT/EV3"=w1128:T6)  [unwired: 2 in]
      n256 = xnode "Move Servos"("Position 6"=u8 8, "Position 5"=u8 237, "Position 4"=u8 40, "Position 3"=u8 7, "Position 2"=u8 0, "Position 1"=u8 220, "Motors"=w1136, "NXT/EV3"=w1128) -> ("NXT/EV3"=w1127:T6)
      n257 = xnode "Motors"() -> ("Motor"=w1182:cluster{"TetrixDCMotor":T3, "TetrixDCMotor":T3})
      n258 = call-poly <vilib>:"PolyWait.vi"("Time (1 sec)"=sgl 1.0, "NXT/EV3"=w1127) -> ("NXT/EV3"=w1138:T6)  [unwired: 2 in]
      n259 = xnode "Move Motors"("Power/Speed 2"=i8 50, "Power/Speed 1"=i8 50, "Motors"=w1182, "NXT/EV3"=w1138) -> ("NXT/EV3"=w1185:T6)
      n260 = call-poly <vilib>:"PolyWait.vi"("Centimeters (40)"=sgl 8.0, "NXT/EV3"=w1185, "Port (Port 1)"=w1169) -> ("NXT/EV3"=w1183:T6)  [unwired: 1 in]
      n261 = xnode "Motors"() -> ("Motor"=w1149:cluster{"TetrixDCMotor":T3, "TetrixDCMotor":T3})
      n262 = xnode "Stop Motors"("Motors"=w1182, "NXT/EV3"=w1183) -> ("NXT/EV3"=w1158:T6)
      n263 = call-poly <vilib>:"PolyWait.vi"("Time (1 sec)"=sgl 1.0, "NXT/EV3"=w1158) -> ("NXT/EV3"=w1141:T6)  [unwired: 2 in]
      n264 = xnode "Move Motors"("Power/Speed 2"=i8 -5, "Power/Speed 1"=i8 -5, "Motors"=w1149, "NXT/EV3"=w1141) -> ("NXT/EV3"=w1155:T6)
      n265 = call-poly <vilib>:"PolyWait.vi"("Centimeters (50)"=sgl 6.0, "NXT/EV3"=w1155, "Port (Port 1)"=w1152) -> ("NXT/EV3"=w1153:T6)  [unwired: 1 in]
      n266 = xnode "Motors"() -> ("Motor"=w1143:cluster{"TetrixDCMotor":T3, "TetrixDCMotor":T3})
      n267 = xnode "Stop Motors"("Motors"=w1149, "NXT/EV3"=w1153) -> ("NXT/EV3"=w1147:T6)
      n268 = call-poly <vilib>:"PolyWait.vi"("Time (1 sec)"=sgl 1.0, "NXT/EV3"=w1147) -> ("NXT/EV3"=w1146:T6)  [unwired: 2 in]
      n269 = xnode "Move Motors"("Power/Speed 2"=i8 5, "Power/Speed 1"=i8 5, "Motors"=w1143, "NXT/EV3"=w1146) -> ("NXT/EV3"=w1145:T6)
      n270 = call-poly <vilib>:"PolyWait.vi"("Time (1 sec)"=sgl 1.0, "NXT/EV3"=w1145) -> ("NXT/EV3"=w1144:T6)  [unwired: 2 in]
      n271 = xnode "Motors"() -> ("Motor"=w1178:T3)
      n272 = xnode "Motors"() -> ("Motor"=w1174:T3)
      n273 = xnode "Stop Motors"("Motors"=w1143, "NXT/EV3"=w1144) -> ("NXT/EV3"=w1140:T6)
      n274 = call-poly <vilib>:"PolyWait.vi"("Time (1 sec)"=sgl 1.5, "NXT/EV3"=w1140) -> ("NXT/EV3"=w1172:T6)  [unwired: 2 in]
      n275 = xnode "Move Motors"("Power/Speed 1"=i8 10, "Motors"=w1178, "NXT/EV3"=w1172) -> ("NXT/EV3"=w1180:T6)
      n276 = xnode "Move Motors"("Power/Speed 1"=i8 10, "Motors"=w1174, "NXT/EV3"=w1172) -> ("NXT/EV3"=w1175:T6)
      n277 = xnode "Motors"() -> ("Sensor"=w1171:T7)
      n278 = xnode "Motors"() -> ("Sensor"=w1170:T7)
      n279 = call-poly <vilib>:"PolyWait.vi"("NXT/EV3"=w1180, "Port (Port 1)"=w1170) -> ("NXT/EV3"=w1179:T6)  [unwired: 2 in]
      n280 = call-poly <vilib>:"PolyWait.vi"("NXT/EV3"=w1175, "Port (Port 1)"=w1171) -> ("NXT/EV3"=w1173:T6)  [unwired: 2 in]
      n281 = xnode "Motors"() -> ("Motor"=w1166:cluster{"TetrixDCMotor":T3, "TetrixDCMotor":T3})
      n282 = xnode "Stop Motors"("Motors"=w1178, "NXT/EV3"=w1179) -> ()  [unwired: 1 out]
      n283 = xnode "Stop Motors"("Motors"=w1174, "NXT/EV3"=w1173) -> ("NXT/EV3"=w1168:T6)
      n284 = call-poly <vilib>:"PolyWait.vi"("Time (1 sec)"=sgl 2.0, "NXT/EV3"=w1168) -> ("NXT/EV3"=w1164:T6)  [unwired: 2 in]
      n285 = xnode "Move Motors"("Power/Speed 2"=i8 -5, "Power/Speed 1"=i8 -5, "Motors"=w1166, "NXT/EV3"=w1164) -> ("NXT/EV3"=w1161:T6)
      n286 = call-poly <vilib>:"PolyWait.vi"("Time (1 sec)"=sgl 0.2, "NXT/EV3"=w1161) -> ("NXT/EV3"=w1160:T6)  [unwired: 2 in]
      n287 = xnode "Stop Motors"("Motors"=w1166, "NXT/EV3"=w1160) -> ("NXT/EV3"=w1137:T6)
    }
  }
  n288 = flat-sequence {
    tunnel: w1 -> [w1286]
    frame #0 {
      w1289 = T7 2 items=["Port 1", "Port 2", "Port 3", "Port 4"] ("Port (Port 1)")
      w1317 = T7 2 items=["Port 1", "Port 2", "Port 3", "Port 4"] ("Port (Port 1)")
      n289 = xnode "Motors"() -> ("Motor"=w1336:cluster{"TetrixDCMotor":T3, "TetrixDCMotor":T3})
      n290 = call-poly <vilib>:"PolyWait.vi"("Time (1 sec)"=sgl 1.5, "NXT/EV3"=w1286) -> ("NXT/EV3"=w1285:T6)  [unwired: 2 in]
      n291 = xnode "Move Motors"("Power/Speed 2"=i8 -100, "Power/Speed 1"=i8 -100, "Motors"=w1336, "NXT/EV3"=w1285) -> ("NXT/EV3"=w1339:T6)
      n292 = call-poly <vilib>:"PolyWait.vi"("Time (1 sec)"=sgl 2.0, "NXT/EV3"=w1339) -> ("NXT/EV3"=w1337:T6)  [unwired: 2 in]
      n293 = xnode "Motors"() -> ("Motor"=w1330:cluster{"TetrixDCMotor":T3, "TetrixDCMotor":T3})
      n294 = xnode "Stop Motors"("Motors"=w1336, "NXT/EV3"=w1337) -> ("NXT/EV3"=w1328:T6)
      n295 = call-poly <vilib>:"PolyWait.vi"("Time (1 sec)"=sgl 1.5, "NXT/EV3"=w1328) -> ("NXT/EV3"=w1327:T6)  [unwired: 2 in]
      n296 = xnode "Move Motors"("Power/Speed 2"=i8 -100, "Power/Speed 1"=i8 -100, "Motors"=w1330, "NXT/EV3"=w1327) -> ("NXT/EV3"=w1333:T6)
      n297 = call-poly <vilib>:"PolyWait.vi"("Time (1 sec)"=sgl 1.0, "NXT/EV3"=w1333) -> ("NXT/EV3"=w1331:T6)  [unwired: 2 in]
      n298 = xnode "Motors"() -> ("Motor"=w1320:cluster{"TetrixDCMotor":T3, "TetrixDCMotor":T3})
      n299 = xnode "Stop Motors"("Motors"=w1330, "NXT/EV3"=w1331) -> ("NXT/EV3"=w1325:T6)
      n300 = call-poly <vilib>:"PolyWait.vi"("Time (1 sec)"=sgl 1.0, "NXT/EV3"=w1325) -> ("NXT/EV3"=w1319:T6)  [unwired: 2 in]
      n301 = xnode "Move Motors"("Power/Speed 2"=i8 -5, "Power/Speed 1"=i8 -5, "Motors"=w1320, "NXT/EV3"=w1319) -> ("NXT/EV3"=w1322:T6)
      n302 = call-poly <vilib>:"PolyWait.vi"("Color (Red)"=ColorSensorColors."Black", "NXT/EV3"=w1322, "Port (Port 1)"=w1317) -> ("NXT/EV3"=w1321:T6)  [unwired: 1 in]
      n303 = xnode "Motors"() -> ("Motor"=w1311:cluster{"TetrixDCMotor":T3, "TetrixDCMotor":T3})
      n304 = xnode "Stop Motors"("Motors"=w1320, "NXT/EV3"=w1321) -> ("NXT/EV3"=w1290:T6)
      n305 = call-poly <vilib>:"PolyWait.vi"("Time (1 sec)"=sgl 0.5, "NXT/EV3"=w1290) -> ("NXT/EV3"=w1300:T6)  [unwired: 2 in]
      n306 = xnode "Move Motors"("Power/Speed 2"=i8 5, "Power/Speed 1"=i8 5, "Motors"=w1311, "NXT/EV3"=w1300) -> ("NXT/EV3"=w1312:T6)
      n307 = call-poly <vilib>:"PolyWait.vi"("Color (Red)"=ColorSensorColors."Black", "NXT/EV3"=w1312, "Port (Port 1)"=w1289) -> ("NXT/EV3"=w1313:T6)  [unwired: 1 in]
      n308 = xnode "Motors"() -> ("Motor"=w1302:cluster{"TetrixDCMotor":T3, "TetrixDCMotor":T3})
      n309 = xnode "Stop Motors"("Motors"=w1311, "NXT/EV3"=w1313) -> ("NXT/EV3"=w1309:T6)
      n310 = call-poly <vilib>:"PolyWait.vi"("Time (1 sec)"=sgl 1.0, "NXT/EV3"=w1309) -> ("NXT/EV3"=w1306:T6)  [unwired: 2 in]
      n311 = xnode "Move Motors"("Power/Speed 2"=i8 -5, "Power/Speed 1"=i8 -5, "Motors"=w1302, "NXT/EV3"=w1306) -> ("NXT/EV3"=w1304:T6)
      n312 = call-poly <vilib>:"PolyWait.vi"("Time (1 sec)"=sgl 1.23, "NXT/EV3"=w1304) -> ("NXT/EV3"=w1303:T6)  [unwired: 2 in]
      n313 = xnode "Motors"() -> ("Motor"=w1297:T5)
      n314 = xnode "Stop Motors"("Motors"=w1302, "NXT/EV3"=w1303) -> ("NXT/EV3"=w1299:T6)
      n315 = call-poly <vilib>:"PolyWait.vi"("Time (1 sec)"=sgl 1.0, "NXT/EV3"=w1299) -> ("NXT/EV3"=w1291:T6)  [unwired: 2 in]
      n316 = xnode "Move Servos"("Position 6"=u8 8, "Position 5"=u8 80, "Position 4"=u8 40, "Position 3"=u8 7, "Position 2"=u8 0, "Position 1"=u8 230, "Motors"=w1297, "NXT/EV3"=w1291) -> ()  [unwired: 1 out]
    }
  }
